vi "single tp value.vi"(10 "single tp data":string="[Pause Message test]\nExt.Name =;\nOutput string =;#") -> (2 "value":string[](array[string]))   [LabVIEW 2018]
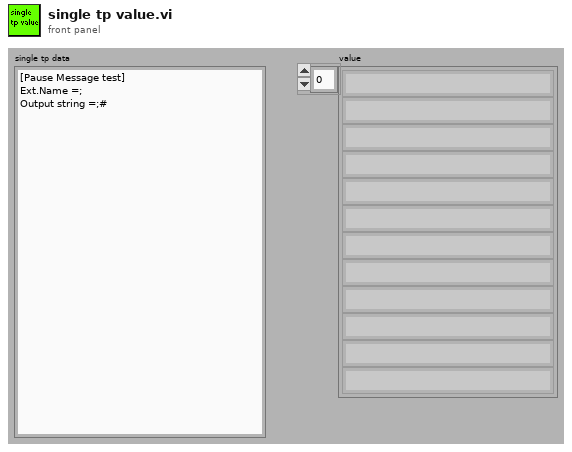
[diagram p1: front panel]
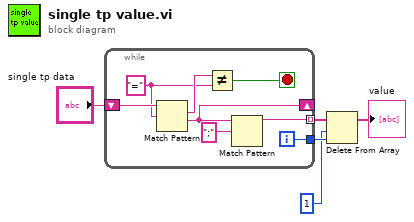
[diagram p0: block diagram]
diagram:
  n1 = while {
    shift-right: [w12] -> _
    shift-left: "single tp data" -> [w13]
    tunnel: [w10] -> w4 mode=indexing
    tunnel: [w6] -> w3
    i -> [w6]
    stop <- w9 stop-if-true
    w7 = "=" ("正则表达式")
    n2 = Match Pattern(string=w13, regular expression=w7) -> (match substring=w8:string, after substring=w12:string)  [unwired: 3 out]
    n3 = Not Equal?(x=w8, y=w7) -> (x != y?=w9:bool)
    n4 = Match Pattern(string=w12, regular expression=";" ("正则表达式")) -> (before substring=w10:string)  [unwired: 4 out]
  }
  n5 = Delete From Array(array=w4, length=1 ("长度"), index=w3) -> (array with subset deleted=→"value":string[])  [unwired: 1 out]
